vi "Self Test.vi"(8 "error in (no error)":errorcluster, 11 "Session Handle":refnum<k15>) -> (0 "error out":errorcluster, 1 "Self Test Message":string, 2 "Self Test Result":i16, 3 "Session Handle Out":refnum<k15>)   [LabVIEW 2026, in "PXI4072.lvlib"]
uses:
  PXI4072.lvlib
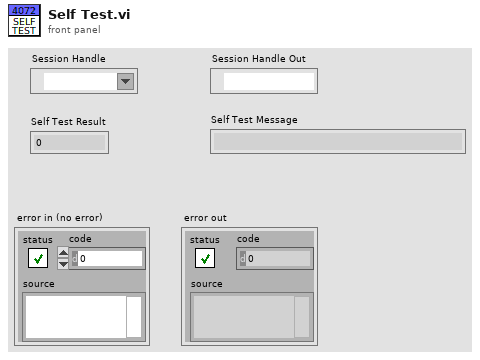
[diagram p1: front panel]
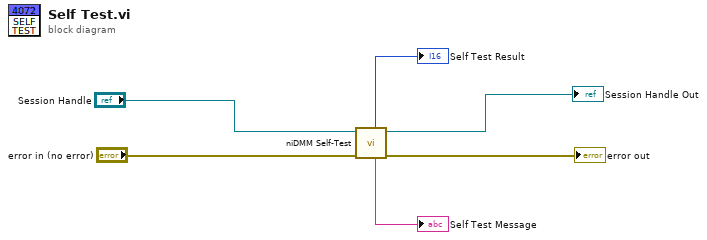
[diagram p0: block diagram]
diagram:
  n1 = call <instrlib>:"niDMM Self-Test.vi"("error in (no error)"="error in (no error)", "instrument handle"="Session Handle") -> ("error out"=→"error out":errorcluster, "instrument handle out"=→"Session Handle Out":refnum<k15>, "Self Test Message"=→"Self Test Message":string, "Self Test Result"=→"Self Test Result":i16)  [unwired: 6 in]
